vi "Photodetector DAQ using PXI5171.vi"() -> ()   [LabVIEW 2018]
uses:
  <instrlib>/niScope/Controls/niScope array measurement.ctl
  <instrlib>/niScope/Controls/niScope trigger source digital.ctl
  <vilib>/Utility/error.llb/DialogType.ctl
  <vilib>/Analysis/8numeric.llb/1D Numeric Integration.vi
  <instrlib>/niScope/Configure/Trigger/niScope Configure Trigger Digital.vi
  <instrlib>/niScope/Configure/Trigger/niScope Configure Trigger Edge.vi
  <instrlib>/niScope/Acquire/Fetch/niScope Multi Fetch Binary 16.vi
  <instrlib>/niScope/Acquire/niScope Get Scaling Coefficients.vi
  <instrlib>/niScope/Measurements/niScope Fetch Measurement.vi
  <instrlib>/niScope/Measurements/niScope Multi Fetch Array Measurement Cluster.vi
  <vilib>/Analysis/NI_AALPro.lvlib
panel:
  out "Loop iteration time":dbl
  in  "PMT Channel":i32
  in  "Photodiode channel":i32=1
  in  "Min. Sample Rate":dbl=20000.0 caption="Sample Rate" format="%#_6p"
  in  "Min Record Length":i32=400 caption="Record Length"
  in  "Trigger type":enum32{"Analog edge", "Digital edge"}(tab) caption="tab control"
  in  "Trigger delay 2":dbl caption="Trigger delay (s)" step=0.1 format="%_3g"
  in  "Trigger Slope":i32(ring) items=["Positive", "Negative"]
  in  "Trigger level (V)":dbl step=0.1 format="%_3g"
  in  "Trigger source":string(combo)="0"
  in  "Trigger Slope 2":i32(ring) caption="Trigger Slope" items=["Positive", "Negative"]
  in  "Trigger delay (V) 2":dbl caption="Trigger delay (s)" step=0.1 format="%_3g"
  in  "trigger source":T1="VAL_RTSI_0"
  in  "Channel settings":T2(array[cluster])=[{"Channel(s)"="0", "Vertical Range (V)"="", "Vertical Coupling"=1}] {"Vertical Coupling" items=["AC", "DC", "Ground"]}
  out "Minimum of absorption signal":dbl[](graph)
  out "Integral of PMT signal":dbl[](graph)
  in  "Save data?":bool
  in  "Save file path":path=path "test.h5"
  out "Error message":string=" INSTRUCTIONS:\r\rNormal Use:  When using subVIs that incorporate the error in/error out (or error I/O) structure, place this handler where you want to inform the user of an error, typically at the end of the I/O data path, as the last action of the program.  If the error in error? is ERROR, the handler creates a message describing the error and its source.  If the type of dialog = 1 (default), the message is displayed to the user, who can only acknowedge it.  If the type = 2, the user can acknowledge the message or abort execution; aborting a program with active I/O is not recommended.  If the type = 0, no message is displayed; this is used to process the error programmatically, and the error out cluster elements are wired to individual terminals for that reason.  \r\rOther Use:\n\r\nlocal testing.  To test the error code of a subVI or function that does not have the error I/O structure, you can wire its error code and a source string to the local error code and error source inputs.  If error in error? indicates no error and error code is not equal to 0, the local code and source are substituted for the error in values, and error? is set TRUE (ERROR)."
  in  "Resource Name":refnum<k15>="DAQ::1"
  out "Waveform From Scope":dbl[][](graph) caption="Waveform from Scope"
  in  "Stop":bool caption="stop"
  in  "Tab Control":T3(tab) caption="tab control"
  in  "Scalar measurements":T4(array[cluster]) {"Measurement" items=["None"=4000, "Frequency"=2, "Average Frequency"=1016, "FFT Frequency"=1008, "Period"=3, "Average Period"=1015, "Rise Time"=0, "Fall Time"=1, "Rising Slew Rate"=1010, "Falling Slew Rate"=1011, "Overshoot"=18, "Preshoot"=19, "Voltage RMS"=4, "Voltage Cycle RMS"=16, "AC Estimate"=1012, "FFT Amplitude"=1009, "Voltage Average"=10, "Voltage Cycle Average"=17, "DC Estimate"=1013, "Voltage Max"=6, "Voltage Min"=7, "Voltage Peak-to-Peak"=5, "Voltage High"=8, "Voltage Low"=9, "Voltage Amplitude"=15, "Voltage Top"=1007, "Voltage Base"=1006, "Voltage Base-to-Top"=1017, "Negative Width"=11, "Positive Width"=12, "Negative Duty Cycle"=13, "Positive Duty Cycle"=14, "Integral"=1005, "Area"=1003, "Cycle Area"=1004, "Time Delay"=1014, "Phase Delay"=1018, "Low Ref Volts"=1000, "Mid Ref Volts"=1001, "High Ref Volts"=1002, "Volt. Hist. Mean"=2000, "Volt. Hist. Stdev"=2001, "Volt. Hist. Median"=2003, "Volt. Hist. Mode"=2010, "Volt. Hist. Max"=2005, "Volt. Hist. Min"=2006, "Volt. Hist. Peak-to-Peak"=2002, "Volt. Hist. Mean + Stdev"=2007, "Volt. Hist. Mean + 2 Stdev"=2008, "Volt. Hist. Mean + 3 Stdev"=2009, "Volt. Hist. Hits"=2004, "Volt. Hist. New Hits"=2011, "Time Hist. Mean"=3000, "Time Hist. Stdev"=3001, "Time Hist. Median"=3003, "Time Hist. Mode"=3010, "Time Hist. Max"=3005, "Time Hist. Min"=3006, "Time Hist. Peak-to-Peak"=3002, "Time Hist. Mean + Stdev"=3007, "Time Hist. Mean + 2 Stdev"=3008, "Time Hist. Mean + 3 Stdev"=3009, "Time Hist. Hits"=3004, "Time Hist. New Hits"=3011]}
  in  "Channels":string
  in  "Array Measurement":T5=4019 items=["None"=4000, "Last Acq. Histogram"=4001, "Multi Acq. Voltage Histogram"=4004, "Multi Acq. Time Histogram"=4005, "Multi Acq. Average"=4016, "Polynomial Interpolation"=4011, "Array Integral"=4006, "Derivative"=4007, "Inverse"=4008, "Multiply Channels"=4012, "Add Channels"=4013, "Subtract Channels"=4014, "Divide Channels"=4015, "Array Offset"=4025, "Array Gain"=4026, "Hanning Window"=4009, "Flat Top Window"=4010, "Hamming Window"=4020, "Triangle Window"=4023, "Blackman Window"=4024, "FIR Windowed Filter"=4021, "Bessel IIR Filter"=4022, "Butterworth IIR Filter"=4017, "Chebyshev IIR Filter"=4018, "FFT Phase Spectrum"=4002, "FFT Amp. Spectrum (Volts RMS)"=4003, "FFT Amp. Spectrum (dB)"=4019]
  out "array measurement result":T6(graph) caption="Array Measurement Result"
  # "Photodetector DAQ"
  # "Trigger settings"
  # "Using loop iteration time to check \nthe program isn't missing triggers"
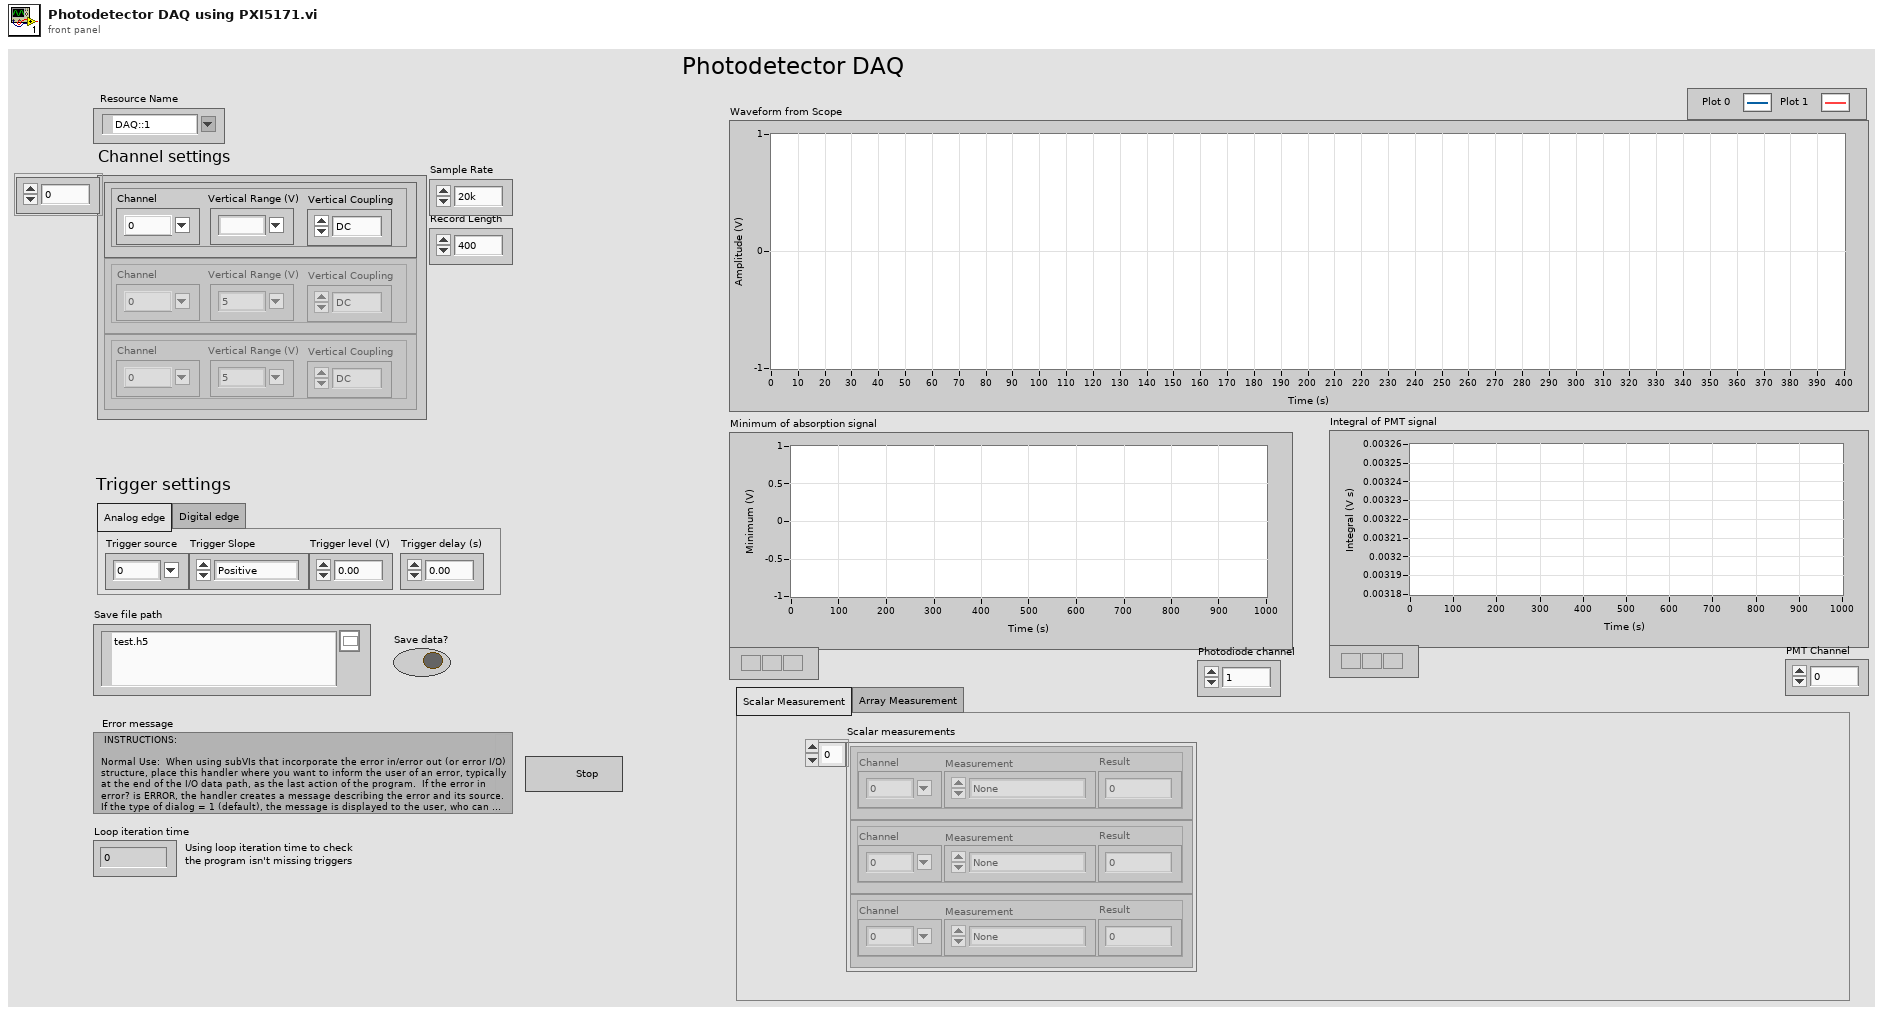
[diagram p1: front panel]
types:
  T1 = typedef "niScope trigger source digital.ctl" = string
  T2 = cluster{"Channel(s)":string, "Vertical Range (V)":string, "Vertical Coupling":i32}[]
  T3 = enum32{"Scalar Measurement", "Array Measurement"}
  T4 = cluster{"Measurement":i32, "Channel":string, "Result":dbl}[]
  T5 = typedef "niScope array measurement.ctl" = i32
  T6 = cluster{"relativeInitialX":dbl, "xIncrement":dbl, "measWfm":dbl[]}[]
  T7 = typedef "HDF5 Ref.ctl" = refnum<k1>
  T8 = typedef "DialogType.ctl" = u16
  T9 = cluster{"offset":dbl, "gain":dbl, "reserved 1":dbl, "reserved 2":dbl}[]
  T10 = cluster{"Measurement":i32, "Channel":string, "result":dbl}
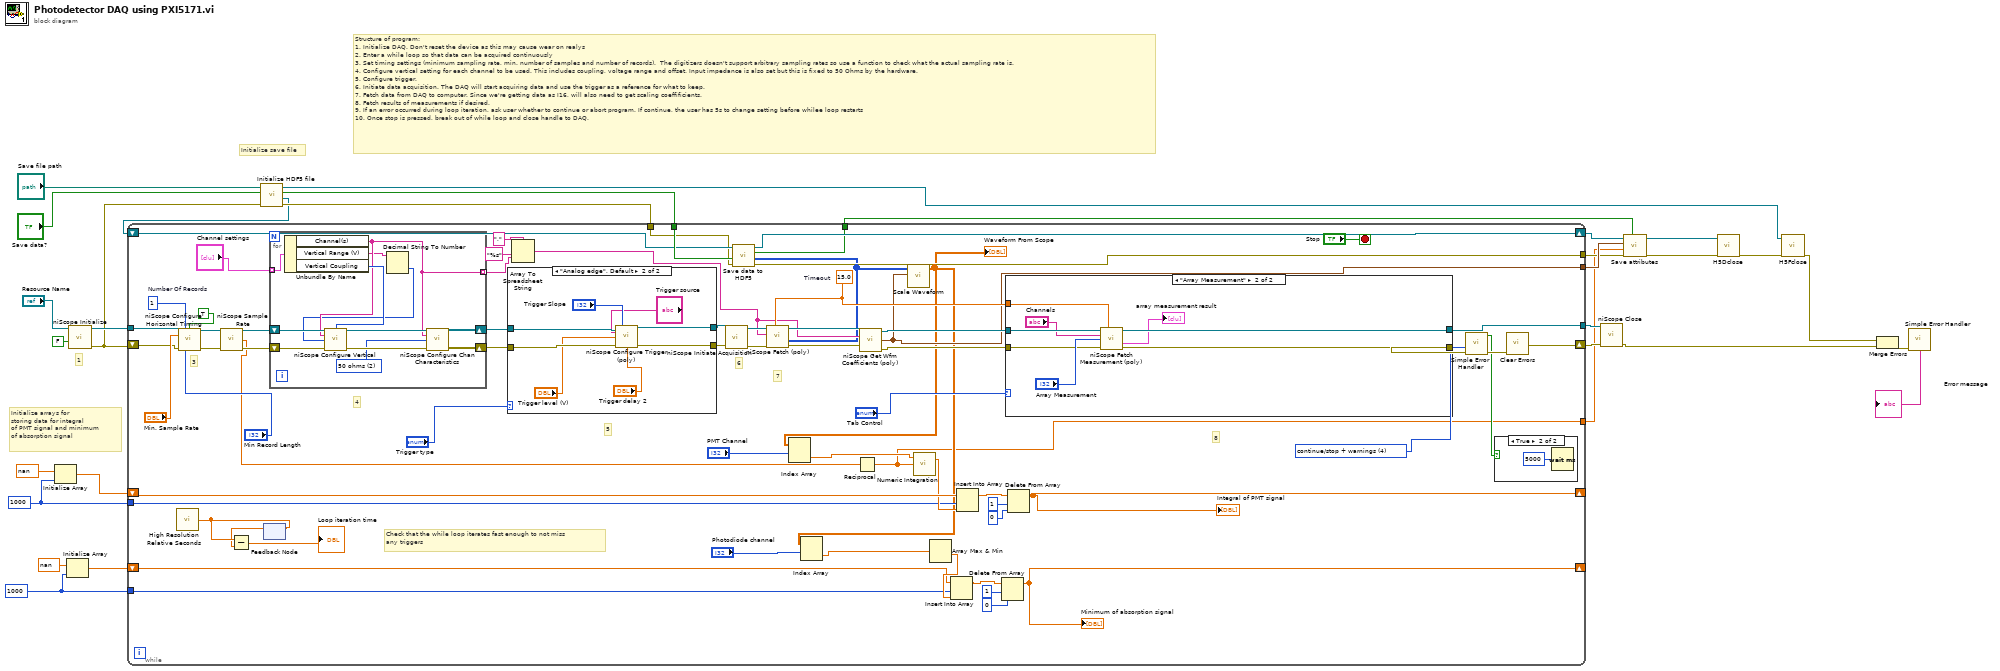
[diagram p0: block diagram]
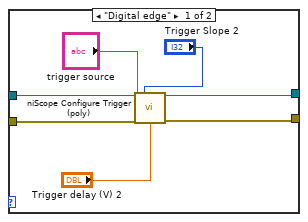
[diagram p2: hidden frame]
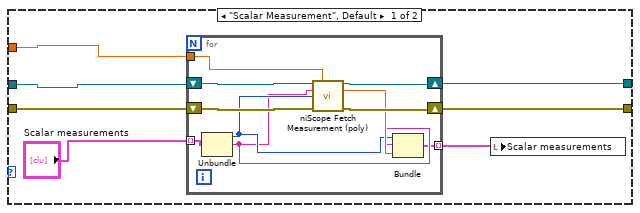
[diagram p4: hidden frame]
diagram:
  w12 = 1000 ("dimension size")
  w15 = 1000 ("dimension size")
  # "1"
  # "Structure of program:\n1. Initialize DAQ. Don't reset the device as this may cause wear on realys\n2. Enter a while loop so that data can be acquired continuously\n3. Set timing settings (minimum sampling rate, min. number of samples and number of records).  The digitizers doesn't support arbitrary sampling rates so use a function to check what the actual sampling rate is.\n4. Configure vertical setting for each channel to be used. This includes coupling, voltage range and offset. Input impedance is also set but this is fixed to 50 Ohms by the hardware.\n5. Configure trigger. \n6. Initiate data acquisition. The DAQ will start acquiring data and use the trigger as a reference for what to keep.\n7. Fetch data from DAQ to computer. Since we're getting data as I16, will also need to get scaling coeffificients.\n8. Fetch results of measurements if desired.\n9. If an error occurred during loop iteration, ask user whether to continue or abort program. If continue, the user has 5s to change setting before whilee loop restarts\n10. Once stop is pressed, break out of while loop and close handle to DAQ."
  # "Initialize save file"
  # "Initialize arrays for \nstoring data for integral\nof PMT signal and minimum\nof absorption signal"
  n1 = Initialize Array(nan ("element"), w15) -> (w16:dbl[])
  n2 = Initialize Array(nan ("element"), w12) -> (w13:dbl[])
  n3 = call <instrlib>:"niScope Initialize.vi"("resource name"="Resource Name", "reset device"=FALSE) -> ("instrument handle"=w29:refnum<k15>, "error out"=w19:errorcluster)  [unwired: 12 in]
  n4 = call "Initialize HDF5 file.vi"("error in (no error)"=w19, "Save data? in"="Save data?", "Save data path in"="Save file path") -> ("error out"=w20:errorcluster, "HDF5 Dataset Ref out"=w10:T7, "Save data? out"=w21:bool, "HDF5 Ref out"=w3:T7)  [unwired: 5 in]
  n5 = while {
    tunnel: w29 -> [w64]
    tunnel: [w97] -> w27
    shift-right: [w73] -> w26
    shift-left: w19 -> [w63]
    tunnel: w21 -> [w95]
    tunnel: w20 -> [w93]
    tunnel: [w92] -> w7
    tunnel: w15 -> [w86]
    shift-right: [w85] -> _
    shift-left: w16 -> [w89]
    shift-right: [w79] -> _
    shift-left: w13 -> [w80]
    tunnel: w12 -> [w78]
    shift-right: [w65] -> w8
    shift-left: w10 -> [w94]
    tunnel: [w43] -> w9
    tunnel: [w32] -> w2
    tunnel: [w31] -> w1
    stop <- "Stop" stop-if-true
    w69 = 1  # Number Of Records
    w74 = T8 4 items=["no dialog", "OK message", "continue or stop message", "OK message + warnings", "continue/stop + warnings"] ("type of dialog (OK msg:1)")
    w53 = 15.0  # Timeout
    # "8"
    # "7"
    # "6"
    # "5"
    # "4"
    # "3"
    # "Check that the while loop iterates fast enough to not miss\nany triggers"
    n6 = call <vilib>:"High Resolution Relative Seconds.vi"() -> ("relative seconds"=w35:dbl)
    n7 = call <instrlib>:"niScope Configure Horizontal Timing.vi"("instrument handle"=w64, "number of records"=w69, "enforce realtime"=TRUE ("Enforce Realtime"), "min sample rate"="Min. Sample Rate", "error in"=w63, "min record length"="Min Record Length") -> ("instrument handle out"=w42:refnum<k15>, "error out"=w40:errorcluster)  [unwired: 8 in]
    n8 = call <instrlib>:"niScope Sample Rate.vi"("instrument handle"=w42, "error in"=w40) -> ("instrument handle out"=w41:refnum<k15>, "actual sample rate"=w38:dbl, "error out"=w39:errorcluster)  [unwired: 11 in]
    n9 = feedback-in #1(w35) -> ()
    n10 = feedback #1() -> (w34:dbl)  [unwired: 1 in]
    n11 = Subtract(x=w35, y=w34) -> (x-y=→"Loop iteration time":dbl)
    n12 = for {
      shift-right: [w116] -> w62
      shift-left: w41 -> [w121]
      shift-right: [w117] -> w61
      shift-left: w39 -> [w120]
      tunnel: "Channel settings" -> [w119] mode=indexing
      tunnel: [w115] -> w60 mode=indexing
      w122 = u32 2 items=["1 mega ohm"=0, "50 ohms"=2] ("Input Impedance")
      n13 = Unbundle By Name(w119) -> ("Channel(s)"=w115:string, "Vertical Range (V)"=w114:string, "Vertical Coupling"=w118:i32)
      n14 = Decimal String To Number(string=w114) -> (number=w113:i32)  [unwired: 2 in, 1 out]
      n15 = call <instrlib>:"niScope Configure Vertical.vi"("instrument handle"=w121, "vertical coupling"=w118, "channels"=w115, "vertical range"=w113, "error in"=w120) -> ("instrument handle out"=w123:refnum<k15>, "error out"=w124:errorcluster)  [unwired: 9 in]
      n16 = call <instrlib>:"niScope Configure Chan Characteristics.vi"("instrument handle"=w123, "channels"=w115, "input impedance"=w122, "error in"=w124) -> ("instrument handle out"=w116:refnum<k15>, "error out"=w117:errorcluster)  [unwired: 10 in]
    }
    n17 = case shown="\"Analog edge\", Default" "Trigger type" {
      tunnel: w61 -> [w103 w112]
      tunnel: w62 -> [w104 w111]
      tunnel: [w101 w109] -> w57
      tunnel: [w102 w108] -> w56
      frame "Digital edge" {
        n18 = call-poly <instrlib>:"niScope Configure Trigger (poly).vi"("instrument handle"=w104, "trigger slope"="Trigger Slope 2", "trigger source"="trigger source", "error in"=w103, "trigger delay"="Trigger delay (V) 2") -> ("instrument handle out"=w101:refnum<k15>, "error out"=w102:errorcluster)  [unwired: 9 in]
      }
      frame "Analog edge", Default {
        n19 = call-poly <instrlib>:"niScope Configure Trigger (poly).vi"("instrument handle"=w111, "trigger slope"="Trigger Slope", "trigger source"="Trigger source", "trigger level"="Trigger level (V)", "error in"=w112, "trigger delay"="Trigger delay 2") -> ("instrument handle out"=w109:refnum<k15>, "error out"=w108:errorcluster)  [unwired: 8 in]
      }
    }
    n20 = Array To Spreadsheet String(delimiter (Tab)=",", array=w60, 3:"%s" ("format string")) -> (spreadsheet string=w47:string)
    n21 = call <instrlib>:"niScope Initiate Acquisition.vi"("instrument handle"=w57, "error in"=w56) -> ("instrument handle out"=w55:refnum<k15>, "error out"=w54:errorcluster)  [unwired: 12 in]
    n22 = call-poly <instrlib>:"niScope Fetch (poly).vi"("timeout"=w53, "error in"=w54, "channels"=w47, "instrument handle"=w55) -> ("error out"=w46:errorcluster, "wfm"=w37:i16[][], "instrument handle out"=w48:refnum<k15>)  [unwired: 4 in, 1 out]
    n23 = call "Save data to HDF5.vi"("wfm"=w37, "error in (no error)"=w93, "Save data?"=w95, "HDF5 Dataset Ref"=w94) -> ("error out"=w92:errorcluster, "Save data? out"=w31:bool, "HDF5 Dataset out"=w65:T7)  [unwired: 5 in]
    n24 = Reciprocal(x=w38) -> (1/x=w32:dbl)
    n25 = call-poly <instrlib>:"niScope Get Wfm Coefficients (poly).vi"("instrument handle"=w48, "channels"=w47, "error in"=w46) -> ("instrument handle out"=w45:refnum<k15>, "coefficient info"=w43:T9, "error out"=w44:errorcluster)  [unwired: 10 in]
    n26 = call "Scale Waveform.vi"("coefficient info"=w43, "wfm"=w37) -> ("Array"=w36:dbl[][])  [unwired: 9 in]
    "Waveform From Scope" <- w36
    n27 = Index Array(array=w36, index (row)="PMT Channel") -> (element=w50:dbl[])  [unwired: 1 in]
    n28 = Index Array(array=w36, index (row)="Photodiode channel") -> (element=w49:dbl[])  [unwired: 1 in]
    n29 = call-poly <vilib>:"Numeric Integration.vi"("dt"=w32, "Input Array"=w50) -> ("result"=w87:dbl)  [unwired: 1 in, 1 out]
    n30 = Array Max & Min(array=w49) -> (min value=w81:dbl)  [unwired: 3 out]
    n31 = Insert Into Array(array=w80, index=w78, new element=w81) -> (w82:dbl[])
    n32 = Insert Into Array(array=w89, index=w86, new element=w87) -> (w88:dbl[])
    n33 = Delete From Array(array=w82, length=1, index=0) -> (array with subset deleted=w79:dbl[])  [unwired: 1 out]
    "Minimum of absorption signal" <- w79
    n34 = case shown="\"Array Measurement\"" "Tab Control" {
      tunnel: [w132 w150] -> w97
      tunnel: [w131 w148] -> w76
      tunnel: w45 -> [w130 w146]
      tunnel: w44 -> [w129 w145]
      tunnel: w53 -> [w128 w144]
      frame "Scalar Measurement", Default {
        n35 = for {
          tunnel: "Scalar measurements" -> [w138] mode=indexing
          tunnel: w128 -> [w137]
          shift-right: [w142] -> w132
          shift-left: w130 -> [w140]
          shift-right: [w141] -> w131
          shift-left: w129 -> [w139]
          tunnel: [w133] -> w126 mode=indexing
          n36 = Unbundle(w138) -> ("Measurement"=w135:i32, "Channel"=w134:string)  [unwired: 1 out]
          n37 = call-poly <instrlib>:"niScope Fetch Measurement (poly).vi"("instrument handle"=w140, "timeout"=w137, "channels"=w134, "scalar measurement"=w135, "error in"=w139) -> ("instrument handle out"=w142:refnum<k15>, "result"=w136:dbl, "error out"=w141:errorcluster)  [unwired: 8 in]
          n38 = Bundle("Measurement"=w135, "Channel"=w134, "result"=w136) -> (w133:T10)  [unwired: 1 in]
        }
        n39 = local write "Scalar measurements"(w126) -> ()
      }
      frame "Array Measurement" {
        n40 = call-poly <instrlib>:"niScope Fetch Measurement (poly).vi"("instrument handle"=w146, "timeout"=w144, "channels"="Channels", "array measurement"="Array Measurement", "error in"=w145) -> ("instrument handle out"=w150:refnum<k15>, "meas waveform"=→"array measurement result":T6, "error out"=w148:errorcluster)  [unwired: 7 in, 1 out]
      }
    }
    n41 = Delete From Array(array=w88, length=1, index=0) -> (array with subset deleted=w85:dbl[])  [unwired: 1 out]
    "Integral of PMT signal" <- w85
    n42 = call <vilib>:"Simple Error Handler.vi"("type of dialog (OK msg:1)"=w74, "error in (no error)"=w76) -> ("error?"=w72:bool, "error out"=w75:errorcluster)  [unwired: 3 in, 3 out]
    n43 = case shown="True" w72 {
      frame False {
      }
      frame True {
        n44 = Wait (ms)(milliseconds to wait=u32 5000) -> ()  [unwired: 1 out]
      }
    }
    n45 = call <vilib>:"Clear Errors.vi"("error in (no error)"=w75) -> ("error out"=w73:errorcluster)  [unwired: 5 in, 1 out]
  }
  n46 = call <instrlib>:"niScope Close.vi"("instrument handle"=w27, "error in"=w26) -> ("error out"=w18:errorcluster)  [unwired: 13 in]
  n47 = call "Save attributes.vi"("Save data?"=w1, "error in (no error)"=w7, "Timestep"=w2, "coefficient info"=w9, "Refnum in"=w8) -> ("error out"=w6:errorcluster, "Refnum out"=w4:T7)  [unwired: 5 in]
  n48 = call <vilib>:"H5Dclose.vi"("error in (no error)"=w6, "HDF5 Dataset Ref"=w4) -> ("error out"=w5:errorcluster)  [unwired: 7 in]
  n49 = call <vilib>:"H5Fclose.vi"("error in (no error)"=w5, "HDF5 Ref"=w3) -> ("error out"=w11:errorcluster)  [unwired: 7 in]
  n50 = Merge Errors(w11, w18) -> (w24:errorcluster)
  n51 = call <vilib>:"Simple Error Handler.vi"("error in (no error)"=w24) -> ("message"=→"Error message":string)  [unwired: 4 in, 4 out]
